vi "ButtonEnable.vi"(8 "error in":errorcluster, 10 "Disabled":T1(ring), 11 "Reference":T2) -> (0 "error out":errorcluster)   [LabVIEW 2020]
uses:
  Controls/BR2.ctl
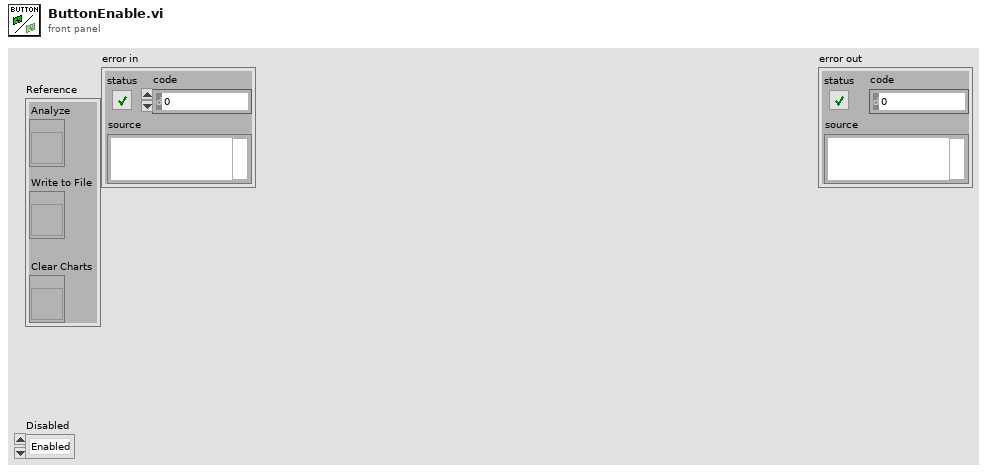
[diagram p1: front panel]
types:
  T1 = enum8{"Enabled", "Disabled", "Disabled and Grayed Out"}
  T2 = typedef "BR2.ctl" = cluster{"Analyze":refnum<vi>, "Write to File":refnum<vi>, "Clear Charts":refnum<vi>}
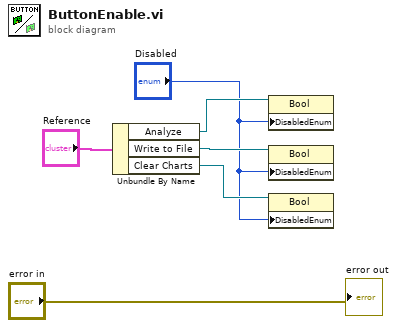
[diagram p0: block diagram]
diagram:
  n1 = Unbundle By Name("Reference") -> ("Analyze"=w3:refnum<vi>, "Write to File"=w4:refnum<vi>, "Clear Charts"=w5:refnum<vi>)
  n2 = property class="Bool"(reference=w3, "DisabledEnum"="Disabled") -> ()  [unwired: 1 in, 2 out]
  n3 = property class="Bool"(reference=w4, "DisabledEnum"="Disabled") -> ()  [unwired: 1 in, 2 out]
  n4 = property class="Bool"(reference=w5, "DisabledEnum"="Disabled") -> ()  [unwired: 1 in, 2 out]
  "error out" <- "error in"
